vi "XML Script - Wire (BD).vi"(3 "destination":string, 4 "source":string, 5 "description":string) -> (0 "destination (dup)":string, 1 "source (dup)":string, 2 "XML Script Command - Wire":string)   [LabVIEW 2017]
uses:
  <vilib>/_script/XML Scripting/XML Script Tag.ctl
  <vilib>/_script/XML Scripting/XML Script Attribute.ctl
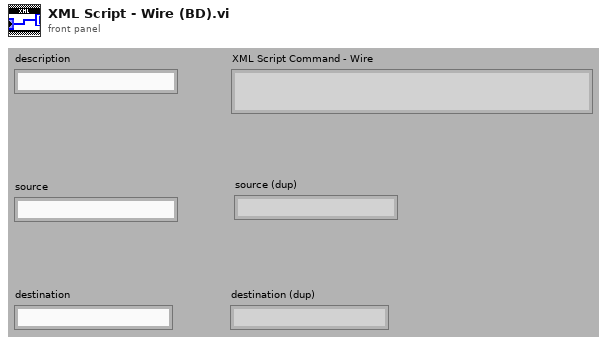
[diagram p1: front panel]
types:
  T1 = typedef "XML Script Attribute.ctl" = enum16{"name", "style", "path", "position", "in", "out", "width", "height", "index", "value", "default", "location", "offset", "typeindex", "size", "source", "destination", "indicator", "type", "controlname", "label", "conpaneidx", "mode", "description", "hasCondTerm", "linkIdentity", "caseselectortype", "concatInputs", "inName", "instantiationpath", "loopCondition", "IndexMode", "formulaInputs", "formulaOutputs", "msnFuncName", "msnIsDynamic", "msnIsODEUserFunction", "ignoreSearchDialog"}
  T2 = typedef "XML Script Tag.ctl" = enum16{"Script", "Function", "SubVI", "GrowableFunction", "Structure", "MultiframeStructure", "Frame", "Tunnel", "ShiftRegister", "Constant", "Control", "Terminal", "Wire", "StaticVIReference", "ControlTerminal", "CompoundArithmetic", "FlatSequence", "FlatSequenceFrame", "MathScriptCallByRef", "BuildArray", "GenericSubVI", "MathScriptNode"}
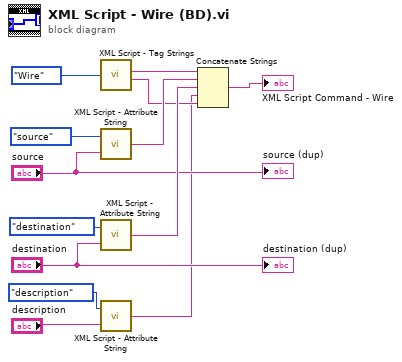
[diagram p0: block diagram]
diagram:
  n1 = call <vilib>:"XML Script - Tag Strings.vi"("XML Script Tag"=XML_Script_Tag."Wire") -> ("XML String - Begin Tag"=w11:string, "XML String - End Tag"=w4:string)  [unwired: 2 in]
  n2 = call <vilib>:"XML Script - Attribute String.vi"("Attribute String"="source", "XML Script Attribute"=XML_Script_Attribute."source") -> ("XML Script - Attribute String"=w9:string)
  n3 = call <vilib>:"XML Script - Attribute String.vi"("Attribute String"="destination", "XML Script Attribute"=XML_Script_Attribute."destination") -> ("XML Script - Attribute String"=w6:string)
  n4 = call <vilib>:"XML Script - Attribute String.vi"("Attribute String"="description", "XML Script Attribute"=XML_Script_Attribute."description") -> ("XML Script - Attribute String"=w2:string)
  n5 = Concatenate Strings(w11, w9, w6, w2, w4) -> (→"XML Script Command - Wire":string)
  "destination (dup)" <- "destination"
  "source (dup)" <- "source"
